vi "Channel Options.vi"() -> ()   [LabVIEW 2020]
uses:
  <vilib>/DAQmx/read.llb/DAQmx Read (Analog 1D Wfm NChan NSamp).vi
  <vilib>/DAQmx/create/channels.llb/DAQmx Create Channel (AI-Voltage-Basic).vi
  <vilib>/DAQmx/configure/timing.llb/DAQmx Timing (Sample Clock).vi
  <vilib>/DAQmx/miscellaneous.llb/DAQmx Fill In Error Info.vi
  <vilib>/measure/maspectr.llb/FFT Spectrum (Mag-Phase) for N Chan.vi
  <vilib>/measure/NI_MAPro.lvlib
  <resource>/objmgr/daqmx.rc
panel:
  in  "Enable Channel":bool[](array[boolean])
  in  "Channel Names":string[](array[string])
  in  "Physical Channels":tag[](array[tag])
  out "Voltage":waveform(dbl)[](graph)
  out "FFT":cluster{"f0":dbl, "df":dbl, "magnitude":dbl[]}[](graph)
  in  "?":enum32{"Input", "Sampling"}(tab)
  in  "Maximum Voltage":dbl=10.0 format="%0.2f"
  in  "Minimum Voltage":dbl=-10.0 format="%0.2f"
  in  "Input Terminal Config.":i32(ring)=10106 items=["Default"=-1, "RSE"=10083, "NRSE"=10078, "Differential"=10106, "Pseudodifferential"=12529]
  in  "# Samples  per Channel":i32=10000
  in  "Requested Rate":dbl=100000.0 format="%0.2f"
  in  "Samples per Channel":i32=1000000
  in  "?":bool
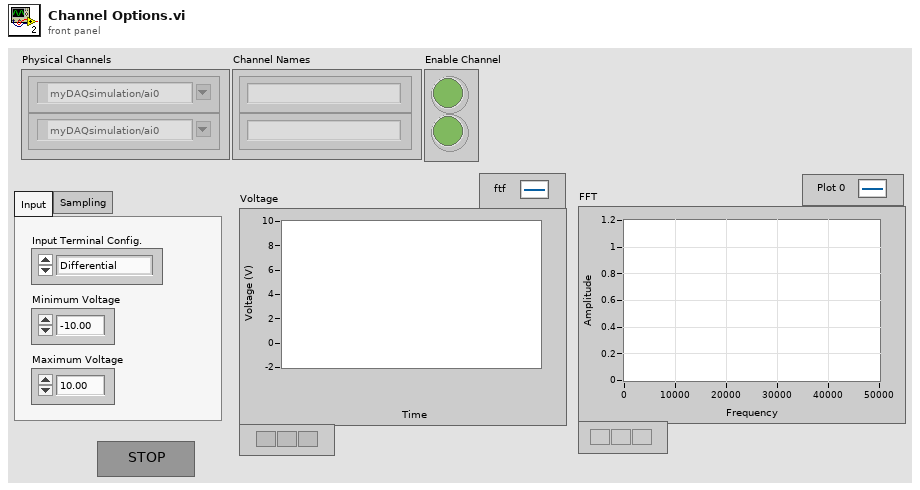
[diagram p1: front panel]
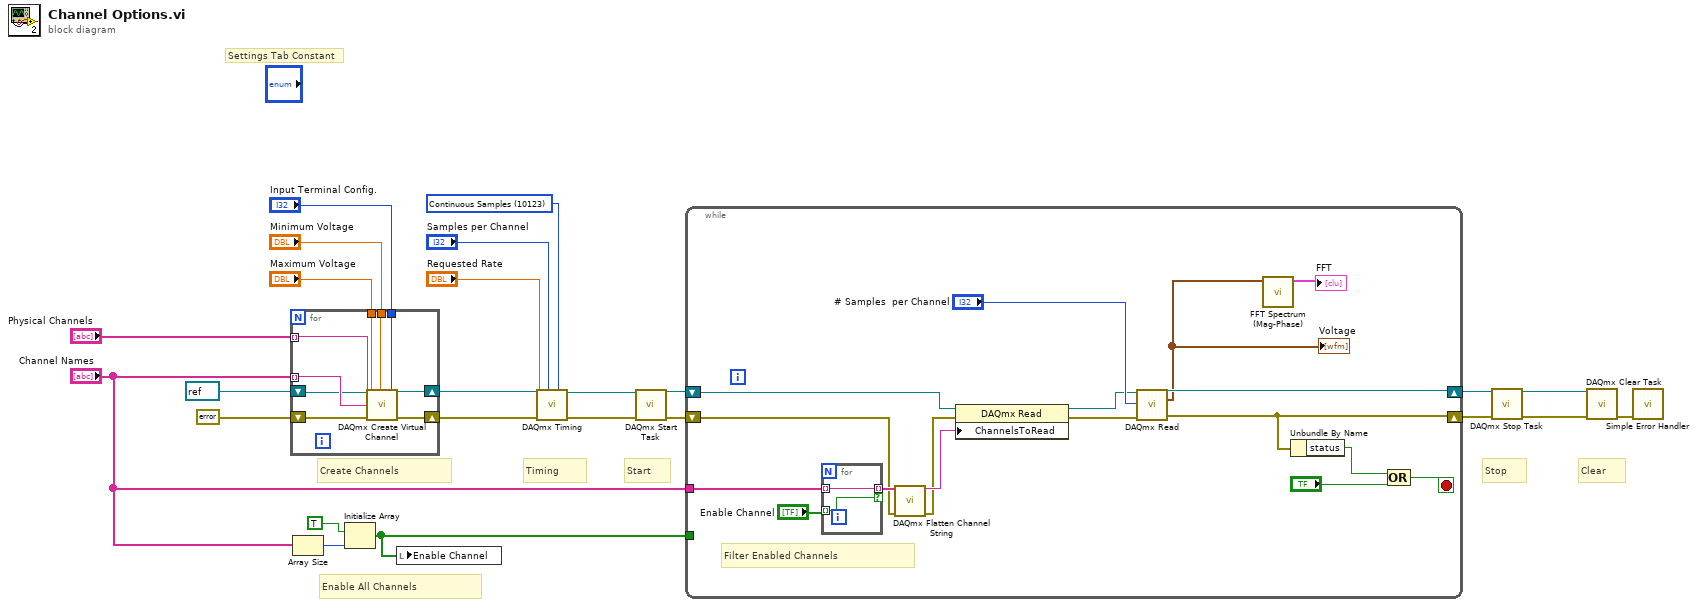
[diagram p0: block diagram]
diagram:
  w14 = 10123 items=["Finite Samples"=10178, "Continuous Samples"=10123, "Hardware Timed Single Point"=12522] ("sample mode")
  # "Enable All Channels"
  # "Clear"
  # "Stop"
  # "Start"
  # "Timing"
  # "Create Channels"
  # "Settings Tab Constant"
  n1 = for {
    tunnel: "Physical Channels" -> [w31] mode=indexing
    tunnel: "Channel Names" -> [w30] mode=indexing
    shift-right: [w32] -> w19
    shift-left: refnum<k21> refnum ("task out") -> [w29]
    shift-right: [w33] -> w23
    shift-left: errorcluster {"status"=FALSE, "code"=0, "source"=""} ("error out") -> [w25]
    tunnel: "Maximum Voltage" -> [w28]
    tunnel: "Minimum Voltage" -> [w27]
    tunnel: "Input Terminal Config." -> [w26]
    n2 = call-poly <vilib>:"DAQmx Create Virtual Channel.vi"("task in"=w29, "maximum value"=w28, "minimum value"=w27, "input terminal configuration"=w26, "physical channels"=w31, "name to assign"=w30, "error in"=w25) -> ("task out"=w32:refnum<k21>, "error out"=w33:errorcluster)  [unwired: 7 in]
  }
  n3 = Array Size(array="Channel Names") -> (size(s)=w4:i32)
  n4 = Initialize Array(TRUE, w4) -> (w2:bool[])
  n5 = local write "Enable Channel"(w2) -> ()
  n6 = call-poly <vilib>:"DAQmx Timing.vi"("task/channels in"=w19, "sample mode"=w14, "samples per channel"="Samples per Channel", "rate"="Requested Rate", "error in"=w23) -> ("task out"=w8:refnum<k21>, "error out"=w7:errorcluster)  [unwired: 9 in]
  n7 = call <vilib>:"DAQmx Start Task.vi"("task/channels in"=w8, "error in"=w7) -> ("task out"=w18:refnum<k21>, "error out"=w22:errorcluster)  [unwired: 12 in]
  n8 = while {
    shift-right: [w49] -> w21
    shift-left: w22 -> [w35]
    shift-right: [w50] -> w17
    shift-left: w18 -> [w41]
    tunnel: w2 -> [_]
    tunnel: "Channel Names" -> [w39]
    stop <- w45 stop-if-true
    # "Filter Enabled Channels"
    n9 = for {
      tunnel: w39 -> [w52] mode=indexing
      tunnel: "Enable Channel" -> [w51] mode=indexing
      tunnel: [w52] -> w37 mode=indexing if=w51
    }
    n10 = call <vilib>:"DAQmx Flatten Channel String.vi"("names in"=w37, "error in"=w35) -> ("names out"=w36:string, "error out"=w34:errorcluster)  [unwired: 12 in]
    n11 = property class="DAQmx Read"(reference=w41, error in=w34, "ChannelsToRead"=w36) -> (reference out=w40:refnum<k21>, error out=w42:errorcluster)
    n12 = call-poly <vilib>:"DAQmx Read.vi"("task/channels in"=w40, "number of samples per channel"="# Samples  per Channel", "error in"=w42) -> ("task out"=w50:refnum<k21>, "data"=w43:waveform(dbl)[], "error out"=w49:errorcluster)  [unwired: 10 in]
    "Voltage" <- w43
    n13 = call-poly <vilib>:"FFT Spectrum (Mag-Phase).vi"("time signals"=w43) -> ("magnitudes"=→"FFT":cluster{"f0":dbl, "df":dbl, "magnitude":dbl[]}[])  [unwired: 6 in, 4 out]
    n14 = Unbundle By Name(w49) -> ("status"=w47:bool)
    n15 = Compound Arithmetic op=OR(w47, "?") -> (w45:bool)
  }
  n16 = call <vilib>:"DAQmx Stop Task.vi"("task/channels in"=w17, "error in"=w21) -> ("task out"=w16:refnum<k21>, "error out"=w20:errorcluster)  [unwired: 12 in]
  n17 = call <vilib>:"DAQmx Clear Task.vi"("task in"=w16, "error in"=w20) -> ("error out"=w9:errorcluster)  [unwired: 13 in]
  n18 = call <vilib>:"Simple Error Handler.vi"("error in (no error)"=w9) -> ()  [unwired: 4 in, 5 out]
